vi "CFN61G_U8-to-B91-92_v1.vi"(11 "U8_Injput":u8[](array[numeric])) -> (2 "CRC_LSB":u8, 3 "CRC_MSB":u8)   [LabVIEW 2017]
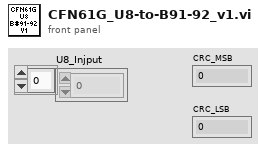
[diagram p1: front panel]
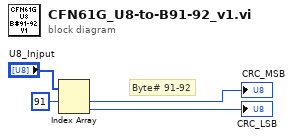
[diagram p0: block diagram]
diagram:
  # "Byte# 91-92"
  n1 = Index Array(array="U8_Injput", index #1=91 ("index")) -> (element #1=→"CRC_MSB":u8, element #2=→"CRC_LSB":u8)  [unwired: 1 in]
